vi "RIO OK Control Loop.vi"   [LabVIEW 2014]
uses:
  <vilib>/Platform/TimedLoop/XDataNode/timing_clust.ctl
  <vilib>/Platform/TimedLoop/XDataNode/nitl_modes.ctl
  <vilib>/Platform/TimedLoop/XDataNode/wakeup.ctl
  Dashboard/SDashLEDs.ctl
  <vilib>/FPGAPlugInAG/sbRIO-9626/niLvFpga_Open_sbRIO-9626.vi
  Global Data.vi
  <vilib>/Utility/error.llb/Error Cluster From Error Code.vi
  <vilib>/rvi/errors/niLvFpgaAdjustHostInterfaceError.vi
  <vilib>/rvi/interface/nirviOpenFPGA/nirviOpenFPGA.xnode
  FPGA Bitfiles/Latest.lvbitx
  <vilib>/Platform/TimedLoop/XDataNode/XDataNode.xnode
  <vilib>/rvi/interface/nirviReadWriteControl/nirviReadWriteControl.xnode
  FPGA Typedef.ctl
  <vilib>/Platform/TimedLoop/XDataNode/XDNodeRunTimeDep.lvlib
  NiFpgaLv.dll
types:
  T1 = typedef "XDNodeRunTimeDep.lvlib/timing_clust.ctl" = cluster{"Expected End [f-1]":u64, "Actual End [f-1]":u64, "Finished Late? [f-1]":bool, "Expected End [i-1]":u64, "Actual End [i-1]":u64, "Finished Late? [i-1]":bool, "Expected Start [i]":u64, "Actual Start [i]":u64, "Expected Start [f]":u64, "Actual Start [f]":u64, "Source Name":string, "Structure Name":string, "Period":i64, "Deadline":i64, "Offset":i64, "Start":i64, "Priority":i32, "Timeout":i32, "Mode":T2, "Wakeup Reason":T3, "Error":errorcluster, "Source Type":string, "Secondary Source Type":string, "Global End Time":u64, "Global Start Time":u64, "Frame Duration":u64, "Iteration Duration":u64, "Assigned CPU":i32, "I/O Scan Engine Mode":u32}
  T2 = typedef "XDNodeRunTimeDep.lvlib/nitl_modes.ctl" = enum32{"No Change", "Process missed periods, maintain original phase", "Discard missed periods, maintain original phase", "Process missed periods, ignore original phase", "Discard missed periods, ignore original phase"}
  T3 = typedef "XDNodeRunTimeDep.lvlib/wakeup.ctl" = enum32{"Normal", "Aborted", "Asynchronous wakeup", "Timing source error", "Timed loop error", "Timeout"}
  T4 = typedef "SDashLEDs.ctl" = cluster{"bGreenLED":bool, "bYellowLED":bool, "bRedLED":bool}
  T5 = typedef "Subsystem Status.ctl" = cluster{"eStatusSeverity":T6, "NValue":sgl, "CMessage":T7, "bNotOK":bool}
  T6 = typedef "Subsystem Status Severity.ctl" = enum16{"Okay", "Short Warning", "Long Warning", "Return to Pits", "Error", "Danger"}
  T7 = typedef "Subsystem Status Message.ctl" = enum16{"ControllerTemperature", "MotorTemperature", "BatteryTemperature", "BatteryLowVoltage", "LVBattery", "sbRIOTemperature", "Precharge", "BSPD", "IMD", "RemoteReturnToPits", "EStopInterrupted", "NoCellComms", "MCOverSpeed", "MCOverCurrent", "MCOverVoltage", "MCInverterOverTemp", "MCDirectionCommand", "MCInverterTimeout", "MCDesatFault", "MCHWOverCurrent", "MCUnderVoltage", "MCCommandMessageLost", "MotorOverTemp", "MCModAOverTemp", "MCModBOverTemp", "MCModCOverTemp", "MCPCBOverTemp", "MCGateDrv1OverTemp", "MCDateDrv2OverTemp", "MCCurrentSensorFault", "MCResolverNotConnected", "ShutdownLatchTripped", "UnknownBMS", "RemoteEmergency"}
  T8 = typedef "FPGA Typedef.ctl" = refnum<k20>
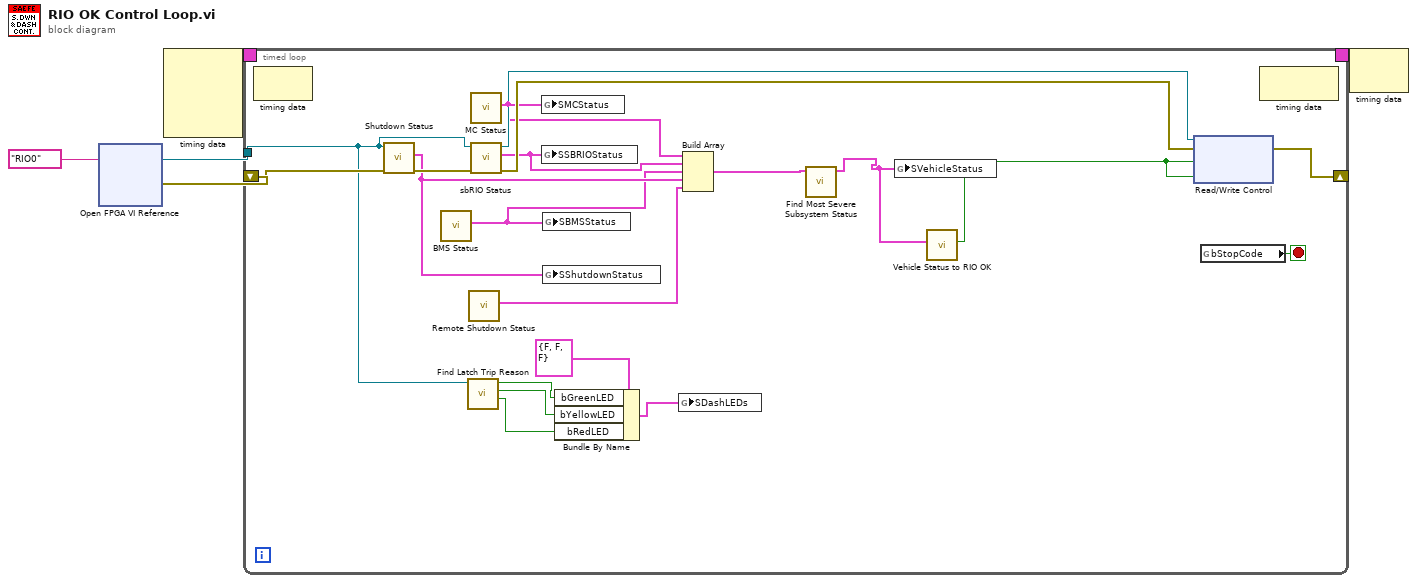
[diagram p0: block diagram]
diagram:
  n1 = xnode "Open FPGA VI Reference"("resource name"=tag "RIO0") -> ("FPGA VI Reference Out"=w2:refnum<k20>, "error out"=w5:errorcluster)  [unwired: 1 in]
  n2 = node-c288() -> (w4:T1)  [unwired: 4 in]
  n3 = timed-loop {
    shift-right: [w22] -> _
    shift-left: w5 -> [w25]
    timing: w4 -> [_]
    timing-out: [_] -> w3
    tunnel: w2 -> [w11]
    stop <- w21 stop-if-true
    n4 = node-c288() -> ()  [unwired: 1 in, 1 out]
    n5 = call "Shutdown Status.vi"("error in"=w25, "FPGA VI Reference In"=w11) -> ("error out"=w24:errorcluster, "Subsystem Status"=w16:T5)  [unwired: 7 in, 1 out]
    n6 = call "BMS Status.vi"() -> ("Subsystem Status"=w14:T5)  [unwired: 11 in]
    n7 = call "Find Latch Trip Reason.vi"("FPGA VI Reference In"=w11) -> ("bBSPDDashLight"=w7:bool, "bIMDDashLight"=w8:bool, "bBMSDashLight"=w9:bool)  [unwired: 8 in]
    n8 = call "Remote Shutdown Status.vi"() -> ("Subsystem Status"=w15:T5)  [unwired: 11 in]
    n9 = call "MC Status.vi"() -> ("Subsystem Status"=w18:T5)  [unwired: 11 in]
    n10 = call "sbRIO Status.vi"("error in (no error)"=w24, "Refnum in"=w11) -> ("error out"=w23:errorcluster, "Subsystem Status"=w17:T5, "Refnum out"=w20:T8)  [unwired: 7 in]
    n11 = global write "Global Data.vi" "SMCStatus"(w18) -> ()
    n12 = global write "Global Data.vi" "SSBRIOStatus"(w17) -> ()
    n13 = global write "Global Data.vi" "SBMSStatus"(w14) -> ()
    n14 = global write "Global Data.vi" "SShutdownStatus"(w16) -> ()
    n15 = Bundle By Name(cluster=T4 {"bGreenLED"=FALSE, "bYellowLED"=FALSE, "bRedLED"=FALSE} ("SDashLEDs"), "bGreenLED"=w9, "bYellowLED"=w8, "bRedLED"=w7) -> (w6:T4)
    n16 = global write "Global Data.vi" "SDashLEDs"(w6) -> ()
    n17 = Build Array(w18, w17, w14, w16, w15) -> (w13:T5[])
    n18 = call "Find Most Severe Subsystem Status.vi"("Array"=w13) -> ("Subystem Status"=w12:T5)  [unwired: 10 in]
    n19 = global write "Global Data.vi" "SVehicleStatus"(w12) -> ()
    n20 = call "Vehicle Status to RIO OK.vi"("Vehicle Status"=w12) -> ("RIO OK"=w19:bool)  [unwired: 10 in]
    n21 = xnode "Read/Write Control"("FPGA VI Reference In"=w20, "error in"=w23, "bSBRIOOK1"=w19, "bSBRIOOK2"=w19) -> ("error out"=w22:errorcluster)  [unwired: 1 out]
    n22 = global read "Global Data.vi" "bStopCode"() -> (w21:bool)
    n23 = node-c288() -> ()  [unwired: 1 in, 1 out]
  }
  n24 = node-c288(w3) -> ()  [unwired: 1 out]
